vi "Receive Event.vi"(8 "error in (no error)":errorcluster, 9 "Event Data":refnum<class "Event Data.lvclass">, 10 "Event Name":string, 11 "Example Sink in":refnum<class "Example Sink.lvclass">) -> (0 "error out":errorcluster, 3 "Example Sink out":refnum<class "Example Sink.lvclass">)   [LabVIEW 2020, in "Example Sink.lvlib" / "Example Sink.lvclass"]
uses:
  Example Sink.lvclass
  Source/Template Source/Event Data/Event Data.lvclass
  Example Sink.lvclass/Example Sink.ctl
  Doublo Array/Doublo Array.lvclass
  Doublo Array/Doublo Array.lvclass/Doublo Array.ctl
  Timestamp/Timestamp.lvclass
  Timestamp/Timestamp.lvclass/Timestamp.ctl
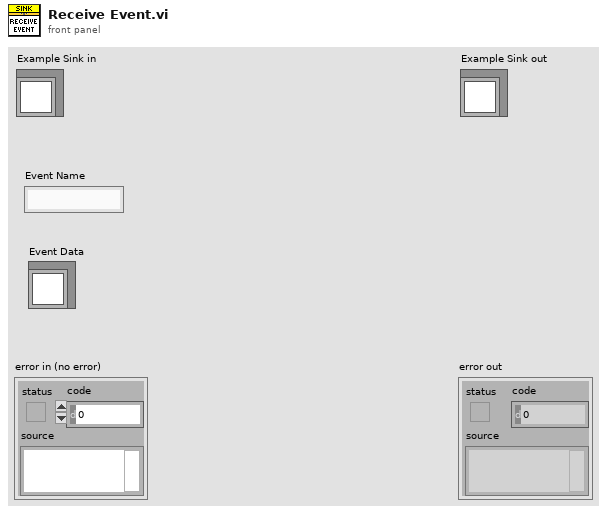
[diagram p1: front panel]
types:
  T1 = typedef "LVDateTimeRec.ctl" = cluster{"fractional second":dbl, "second":i32, "minute":i32, "hour":i32, "day of month":i32, "month":i32, "year":i32, "day of week":i32, "day of year":i32, "DST":i32}
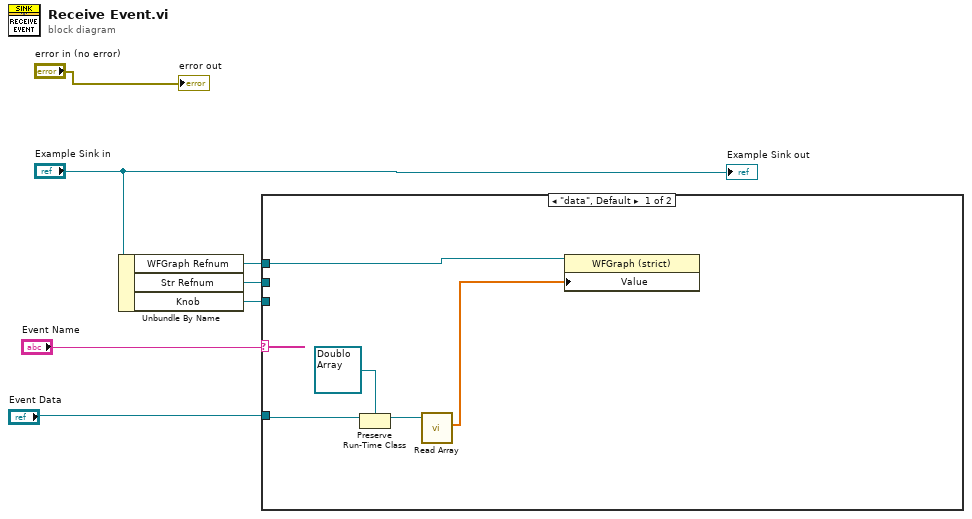
[diagram p0: block diagram]
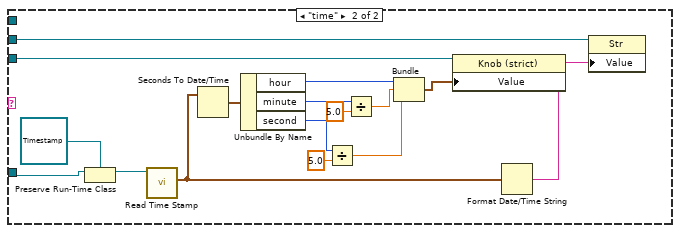
[diagram p2: hidden frame]
diagram:
  n1 = Unbundle By Name("Example Sink in") -> ("WFGraph Refnum"=w5:refnum<vi>, "Str Refnum"=w6:refnum<vi>, "Knob"=w2:refnum<vi>)
  n2 = case shown="\"data\", Default" "Event Name" {
    tunnel: w6 -> [_ w25]
    tunnel: w5 -> [w10 _]
    tunnel: "Event Data" -> [w12 w28]
    tunnel: w2 -> [_ w23]
    frame "data", Default {
      n3 = Preserve Run-Time Class(object in=w12, 2:refnum<class "Doublo Array.lvclass"> refnum ("Example Source.lvlib:Doublo Array.lvclass")) -> (object out=w8:refnum<class "Doublo Array.lvclass">)  [unwired: 1 in, 1 out]
      n4 = call "Read Array.vi"("Doublo Array in"=w8) -> ("Array"=w9:dbl[])  [unwired: 8 in, 2 out]
      n5 = property class="WFGraph (strict)"(reference=w10, "Value"=w9) -> ()  [unwired: 1 in, 2 out]
    }
    frame "time" {
      n6 = Preserve Run-Time Class(object in=w28, 2:refnum<class "Timestamp.lvclass"> refnum ("Example Source.lvlib:time.lvclass")) -> (object out=w26:refnum<class "Timestamp.lvclass">)  [unwired: 1 in, 1 out]
      n7 = call "Read Time Stamp.vi"("time in"=w26) -> ("Time Stamp"=w22:timestamp)  [unwired: 8 in, 2 out]
      n8 = Seconds To Date/Time(time stamp (now)=w22) -> (date time rec=w21:T1)  [unwired: 1 in]
      n9 = Unbundle By Name(w21) -> ("hour"=w20:i32, "minute"=w18:i32, "second"=w14:i32)
      n10 = Divide(x=w14, y=5.0) -> (x/y=w13:dbl)
      n11 = Divide(x=w18, y=5.0) -> (x/y=w17:dbl)
      n12 = Bundle("hour"=w20, w17, w13) -> (w19:cluster{"hour":i32, dbl, dbl})  [unwired: 1 in]
      n13 = property class="Knob (strict)"(reference=w23, "Value"=w19) -> ()  [unwired: 1 in, 2 out]
      n14 = Format Date/Time String(seconds (now)=w22) -> (date/time string=w24:string)  [unwired: 2 in]
      n15 = property class="Str"(reference=w25, "Value"=w24) -> ()  [unwired: 1 in, 2 out]
    }
  }
  "error out" <- "error in (no error)"
  "Example Sink out" <- "Example Sink in"
